vi "_CreateDvr.vi"(10 "DVR":T1) -> (2 "DVR out":T1)   [LabVIEW 2009, in "CellPhone.lvclass"]
doc: "Creates a DVR if the current DVR is invalid."
uses:
  CellPhone.lvclass
  _PrivateDataDvr.ctl
  _PrivateData.ctl
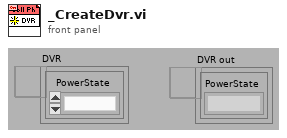
[diagram p1: front panel]
types:
  T1 = typedef "CellPhone.lvclass/_PrivateDataDvr.ctl" = refnum<data-value>
  T2 = typedef "CellPhone.lvclass/_PrivateData.ctl" = cluster{"PowerState":enum16{"Off", "Sleep", "On"}}
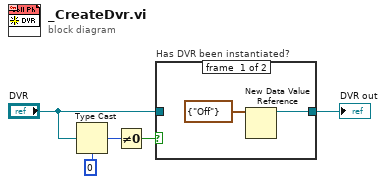
[diagram p0: block diagram]
diagram:
  n1 = Type Cast(type=0, x="DVR") -> (*(type *) &x=w3:i32)
  n2 = Not Equal To 0?(x=w3) -> (x != 0?=w4:bool)
  n3 = case "Has DVR been instantiated?" shown="False" w4 {
    tunnel: "DVR" -> [_ w8]
    tunnel: [w7 w8] -> w1
    frame #0 {
      n4 = New Data Value Reference(data value=T2 {"PowerState"=enum."Off"} ("Private Data")) -> (data value reference=w7:refnum<data-value>)  [unwired: 1 in, 1 out]
    }
    frame #1 {
    }
  }
  "DVR out" <- w1
